vi "프로토콜_테이블.vi"() -> ()   [LabVIEW 2017]
panel:
  in  "data_count":u32=1515870810
  in  "channel_count":u32=1515870810
  in  "data_type":u32=1515870810
  in  "reserved10":i32=1515870810
  in  "reserved9":sgl=1515870800.0
  in  "reserved8":sgl=1515870800.0
  in  "reserved7":sgl=1515870800.0
  in  "reserved6":sgl=1515870800.0
  in  "reserved5":sgl=1515870800.0
  in  "reserved4":sgl=1515870800.0
  in  "reserved3":sgl=1515870800.0
  in  "Longi":dbl=1515870810.0
  in  "Lati":dbl=1515870810.0
  in  "Sec":sgl=1515870800.0
  in  "Minute":i32=1515870810
  in  "Hour":i32=1515870810
  in  "Day":i32=1515870810
  in  "Month":i32=1515870810
  in  "Year":i32=1515870810
  in  "reserved2":i32=1515870810
  in  "reserved1":i32=1515870810
  in  "TVG":i32=1515870810
  in  "Gain":i32=1515870810
  in  "Range":u32=1515870810
  in  "Burst Number":u32=1515870810
  in  "Sampling Freq":u32=1515870810
  in  "Tranducer Freq":u32=1515870810
  in  "Version":u32=1515870810
  in  "MSG ID":i32=1515870810
  in  "packet_length":i32=1515870810
  in  "Start_Flag":i32=1515870810
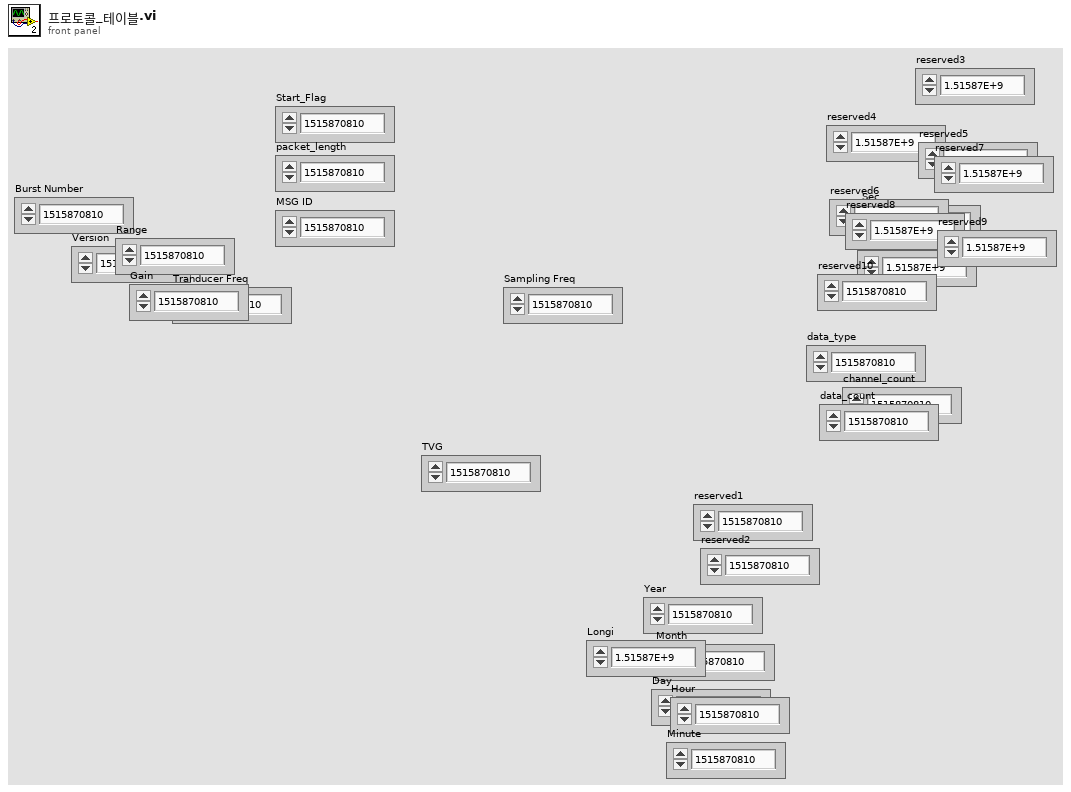
[diagram p1: front panel]
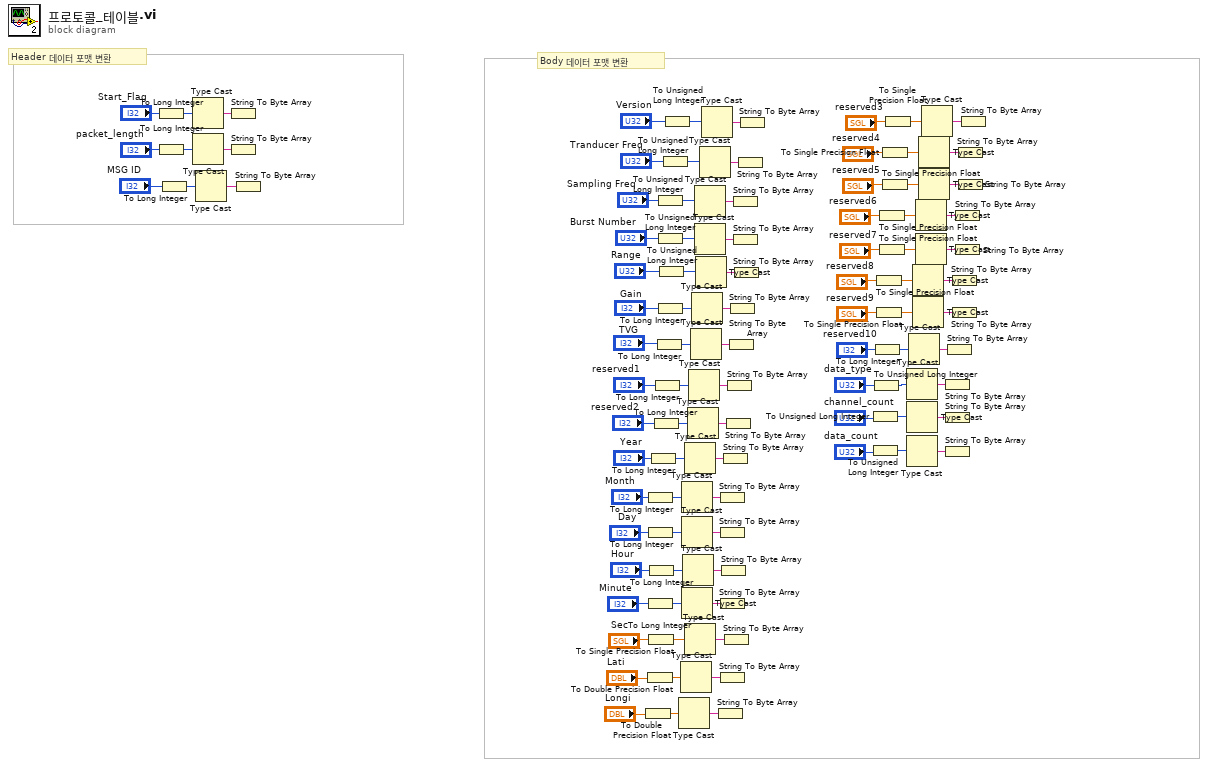
[diagram p0: block diagram]
diagram:
  # "Body 데이터 포맷 변환"
  # "Header 데이터 포맷 변환"
  n1 = To Long Integer(number="Start_Flag") -> (32bit integer=w93:i32)
  n2 = To Long Integer(number="packet_length") -> (32bit integer=w90:i32)
  n3 = To Long Integer(number="MSG ID") -> (32bit integer=w87:i32)
  n4 = Type Cast(x=w93) -> (*(type *) &x=w92:string)  [unwired: 1 in]
  n5 = Type Cast(x=w90) -> (*(type *) &x=w89:string)  [unwired: 1 in]
  n6 = Type Cast(x=w87) -> (*(type *) &x=w86:string)  [unwired: 1 in]
  n7 = String To Byte Array(string=w92) -> ()  [unwired: 1 out]
  n8 = String To Byte Array(string=w89) -> ()  [unwired: 1 out]
  n9 = String To Byte Array(string=w86) -> ()  [unwired: 1 out]
  n10 = To Double Precision Float(number="Longi") -> (double precision float=w34:dbl)
  n11 = To Long Integer(number="Month") -> (32bit integer=w54:i32)
  n12 = To Long Integer(number="Day") -> (32bit integer=w51:i32)
  n13 = To Long Integer(number="Minute") -> (32bit integer=w45:i32)
  n14 = To Double Precision Float(number="Lati") -> (double precision float=w37:dbl)
  n15 = To Long Integer(number="Hour") -> (32bit integer=w48:i32)
  n16 = To Single Precision Float(number="Sec") -> (single precision float=w42:sgl)
  n17 = To Long Integer(number="Year") -> (32bit integer=w57:i32)
  n18 = To Long Integer(number="reserved2") -> (32bit integer=w60:i32)
  n19 = To Long Integer(number="reserved1") -> (32bit integer=w63:i32)
  n20 = To Long Integer(number="TVG") -> (32bit integer=w66:i32)
  n21 = To Unsigned Long Integer(number="Sampling Freq") -> (unsigned 32bit integer=w77:u32)
  n22 = To Unsigned Long Integer(number="Burst Number") -> (unsigned 32bit integer=w74:u32)
  n23 = To Long Integer(number="Gain") -> (32bit integer=w69:i32)
  n24 = To Unsigned Long Integer(number="Range") -> (unsigned 32bit integer=w71:u32)
  n25 = To Unsigned Long Integer(number="Tranducer Freq") -> (unsigned 32bit integer=w80:u32)
  n26 = To Unsigned Long Integer(number="Version") -> (unsigned 32bit integer=w82:u32)
  n27 = Type Cast(x=w34) -> (*(type *) &x=w35:string)  [unwired: 1 in]
  n28 = Type Cast(x=w37) -> (*(type *) &x=w38:string)  [unwired: 1 in]
  n29 = Type Cast(x=w54) -> (*(type *) &x=w53:string)  [unwired: 1 in]
  n30 = Type Cast(x=w51) -> (*(type *) &x=w50:string)  [unwired: 1 in]
  n31 = Type Cast(x=w45) -> (*(type *) &x=w44:string)  [unwired: 1 in]
  n32 = Type Cast(x=w48) -> (*(type *) &x=w47:string)  [unwired: 1 in]
  n33 = Type Cast(x=w57) -> (*(type *) &x=w56:string)  [unwired: 1 in]
  n34 = Type Cast(x=w42) -> (*(type *) &x=w41:string)  [unwired: 1 in]
  n35 = Type Cast(x=w60) -> (*(type *) &x=w59:string)  [unwired: 1 in]
  n36 = Type Cast(x=w63) -> (*(type *) &x=w62:string)  [unwired: 1 in]
  n37 = Type Cast(x=w66) -> (*(type *) &x=w65:string)  [unwired: 1 in]
  n38 = Type Cast(x=w69) -> (*(type *) &x=w68:string)  [unwired: 1 in]
  n39 = Type Cast(x=w77) -> (*(type *) &x=w78:string)  [unwired: 1 in]
  n40 = Type Cast(x=w74) -> (*(type *) &x=w75:string)  [unwired: 1 in]
  n41 = Type Cast(x=w71) -> (*(type *) &x=w72:string)  [unwired: 1 in]
  n42 = Type Cast(x=w80) -> (*(type *) &x=w81:string)  [unwired: 1 in]
  n43 = Type Cast(x=w82) -> (*(type *) &x=w83:string)  [unwired: 1 in]
  n44 = String To Byte Array(string=w35) -> ()  [unwired: 1 out]
  n45 = String To Byte Array(string=w53) -> ()  [unwired: 1 out]
  n46 = String To Byte Array(string=w50) -> ()  [unwired: 1 out]
  n47 = String To Byte Array(string=w44) -> ()  [unwired: 1 out]
  n48 = String To Byte Array(string=w38) -> ()  [unwired: 1 out]
  n49 = String To Byte Array(string=w47) -> ()  [unwired: 1 out]
  n50 = String To Byte Array(string=w56) -> ()  [unwired: 1 out]
  n51 = String To Byte Array(string=w41) -> ()  [unwired: 1 out]
  n52 = String To Byte Array(string=w59) -> ()  [unwired: 1 out]
  n53 = String To Byte Array(string=w62) -> ()  [unwired: 1 out]
  n54 = String To Byte Array(string=w65) -> ()  [unwired: 1 out]
  n55 = String To Byte Array(string=w68) -> ()  [unwired: 1 out]
  n56 = String To Byte Array(string=w78) -> ()  [unwired: 1 out]
  n57 = String To Byte Array(string=w75) -> ()  [unwired: 1 out]
  n58 = String To Byte Array(string=w72) -> ()  [unwired: 1 out]
  n59 = String To Byte Array(string=w81) -> ()  [unwired: 1 out]
  n60 = String To Byte Array(string=w83) -> ()  [unwired: 1 out]
  n61 = To Unsigned Long Integer(number="channel_count") -> (unsigned 32bit integer=w4:u32)
  n62 = To Unsigned Long Integer(number="data_count") -> (unsigned 32bit integer=w1:u32)
  n63 = To Unsigned Long Integer(number="data_type") -> (unsigned 32bit integer=w6:u32)
  n64 = To Long Integer(number="reserved10") -> (32bit integer=w12:i32)
  n65 = To Single Precision Float(number="reserved8") -> (single precision float=w18:sgl)
  n66 = To Single Precision Float(number="reserved9") -> (single precision float=w13:sgl)
  n67 = To Single Precision Float(number="reserved6") -> (single precision float=w24:sgl)
  n68 = To Single Precision Float(number="reserved7") -> (single precision float=w21:sgl)
  n69 = To Single Precision Float(number="reserved4") -> (single precision float=w30:sgl)
  n70 = To Single Precision Float(number="reserved5") -> (single precision float=w27:sgl)
  n71 = To Single Precision Float(number="reserved3") -> (single precision float=w33:sgl)
  n72 = Type Cast(x=w6) -> (*(type *) &x=w9:string)  [unwired: 1 in]
  n73 = Type Cast(x=w4) -> (*(type *) &x=w8:string)  [unwired: 1 in]
  n74 = Type Cast(x=w1) -> (*(type *) &x=w3:string)  [unwired: 1 in]
  n75 = Type Cast(x=w12) -> (*(type *) &x=w11:string)  [unwired: 1 in]
  n76 = Type Cast(x=w18) -> (*(type *) &x=w17:string)  [unwired: 1 in]
  n77 = Type Cast(x=w13) -> (*(type *) &x=w14:string)  [unwired: 1 in]
  n78 = Type Cast(x=w24) -> (*(type *) &x=w23:string)  [unwired: 1 in]
  n79 = Type Cast(x=w21) -> (*(type *) &x=w20:string)  [unwired: 1 in]
  n80 = Type Cast(x=w30) -> (*(type *) &x=w29:string)  [unwired: 1 in]
  n81 = Type Cast(x=w27) -> (*(type *) &x=w26:string)  [unwired: 1 in]
  n82 = Type Cast(x=w33) -> (*(type *) &x=w32:string)  [unwired: 1 in]
  n83 = String To Byte Array(string=w9) -> ()  [unwired: 1 out]
  n84 = String To Byte Array(string=w8) -> ()  [unwired: 1 out]
  n85 = String To Byte Array(string=w3) -> ()  [unwired: 1 out]
  n86 = String To Byte Array(string=w11) -> ()  [unwired: 1 out]
  n87 = String To Byte Array(string=w17) -> ()  [unwired: 1 out]
  n88 = String To Byte Array(string=w14) -> ()  [unwired: 1 out]
  n89 = String To Byte Array(string=w23) -> ()  [unwired: 1 out]
  n90 = String To Byte Array(string=w20) -> ()  [unwired: 1 out]
  n91 = String To Byte Array(string=w29) -> ()  [unwired: 1 out]
  n92 = String To Byte Array(string=w26) -> ()  [unwired: 1 out]
  n93 = String To Byte Array(string=w32) -> ()  [unwired: 1 out]
